vi "Initialize Custom Device Settings.vi"(8 "error in":errorcluster, 10 "Compiled Settings":variant, 11 "Engine Settings in":T2) -> (0 "error out":errorcluster, 1 "ChannelRefs":T1, 3 "Engine Settings out":T2)   [LabVIEW 2026, in "SystemMonitor Engine.lvlib" / "SystemMonitor Engine.lvclass"]
uses:
  SystemMonitor Engine.lvclass
  Types/TargetSettings.ctl
  Shared/GroupedChannelRefs.ctl
  Shared/Compiled.Settings.ctl
  Shared/CustomDeviceSettings.ctl
  Shared/ChannelGroups.ctl
  Shared/GroupSettings.ctl
  Shared/GroupedChannel.ctl
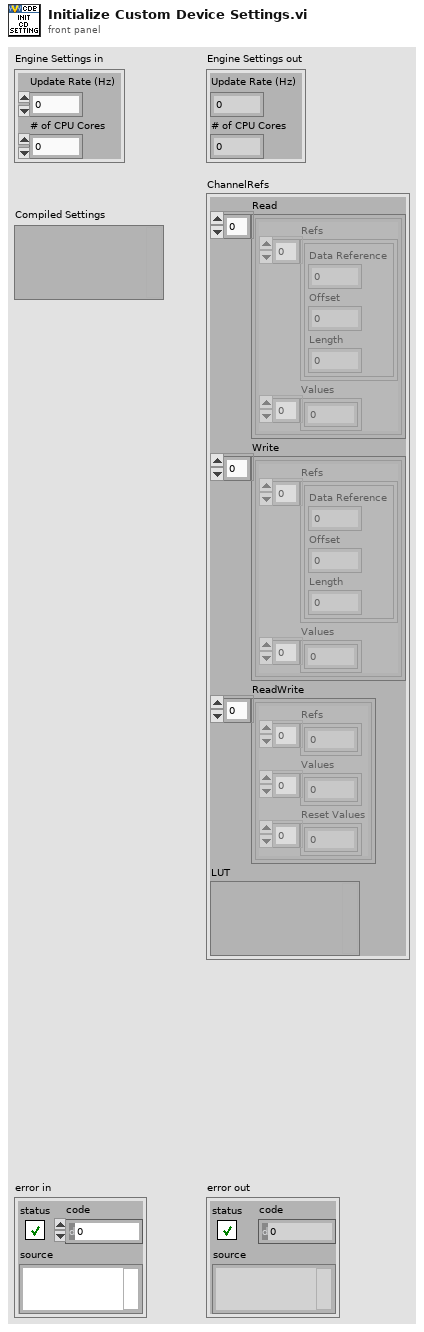
[diagram p1: front panel]
types:
  T1 = typedef "GroupedChannelRefs.ctl" = cluster{"Read":cluster{"Refs":cluster{"Data Reference":i32, "Offset":u64, "Length":u64}[], "Values":dbl[]}[], "Write":cluster{"Refs":cluster{"Data Reference":i32, "Offset":u64, "Length":u64}[], "Values":dbl[]}[], "ReadWrite":cluster{"Refs":i32[], "Values":dbl[], "Reset Values":dbl[]}[], "LUT":variant}
  T2 = typedef "SystemMonitor Engine.lvlib/SystemMonitor Engine.lvclass/TargetSettings.ctl" = cluster{"Update Rate (Hz)":dbl, "# of CPU Cores":i32}
  T3 = typedef "Compiled.Settings.ctl" = cluster{"SystemMonitor":T4, "Channel Groups":T5}
  T4 = typedef "CustomDeviceSettings.ctl" = cluster{"Name":string, "Properties":cluster{"Update Rate (Hz)":dbl, "TargetOS":string, "TargetRate":dbl}, "Sections":cluster{"CPUOverall[]":cluster{"Name":string, "Channels":cluster{"AverageType[]":cluster{"Name":string, "DefaultValue":dbl, "Units":string, "GroupName":string, "Type":string, "Faultable":bool, "Scalable":bool, "ChannelDataReference":i32, "GroupIndex":i32}[], "MaximumType[]":cluster{"Name":string, "DefaultValue":dbl, "Units":string, "GroupName":string, "Type":string, "Faultable":bool, "Scalable":bool, "ChannelDataReference":i32, "GroupIndex":i32}[]}}[], "MemoryUsage[]":cluster{"Name":string, "Channels":cluster{"TotalMemoryType[]":cluster{"Name":string, "DefaultValue":dbl, "Units":string, "GroupName":string, "Type":string, "Faultable":bool, "Scalable":bool, "ChannelDataReference":i32, "GroupIndex":i32}[], "AvailableType[]":cluster{"Name":string, "DefaultValue":dbl, "Units":string, "GroupName":string, "Type":string, "Faultable":bool, "Scalable":bool, "ChannelDataReference":i32, "GroupIndex":i32}[]}}[], "CPU[]":cluster{"Name":string, "Channels":cluster{"TotalType[]":cluster{"Name":string, "DefaultValue":dbl, "Units":string, "GroupName":string, "Type":string, "Faultable":bool, "Scalable":bool, "ChannelDataReference":i32, "GroupIndex":i32}[], "TimeCriticalType[]":cluster{"Name":string, "DefaultValue":dbl, "Units":string, "GroupName":string, "Type":string, "Faultable":bool, "Scalable":bool, "ChannelDataReference":i32, "GroupIndex":i32}[], "TimedStructuresType[]":cluster{"Name":string, "DefaultValue":dbl, "Units":string, "GroupName":string, "Type":string, "Faultable":bool, "Scalable":bool, "ChannelDataReference":i32, "GroupIndex":i32}[], "HighType[]":cluster{"Name":string, "DefaultValue":dbl, "Units":string, "GroupName":string, "Type":string, "Faultable":bool, "Scalable":bool, "ChannelDataReference":i32, "GroupIndex":i32}[], "AboveNormalType[]":cluster{"Name":string, "DefaultValue":dbl, "Units":string, "GroupName":string, "Type":string, "Faultable":bool, "Scalable":bool, "ChannelDataReference":i32, "GroupIndex":i32}[], "NormalType[]":cluster{"Name":string, "DefaultValue":dbl, "Units":string, "GroupName":string, "Type":string, "Faultable":bool, "Scalable":bool, "ChannelDataReference":i32, "GroupIndex":i32}[], "BackgroundType[]":cluster{"Name":string, "DefaultValue":dbl, "Units":string, "GroupName":string, "Type":string, "Faultable":bool, "Scalable":bool, "ChannelDataReference":i32, "GroupIndex":i32}[], "IdleType[]":cluster{"Name":string, "DefaultValue":dbl, "Units":string, "GroupName":string, "Type":string, "Faultable":bool, "Scalable":bool, "ChannelDataReference":i32, "GroupIndex":i32}[], "ISRType[]":cluster{"Name":string, "DefaultValue":dbl, "Units":string, "GroupName":string, "Type":string, "Faultable":bool, "Scalable":bool, "ChannelDataReference":i32, "GroupIndex":i32}[]}}[]}}
  T5 = typedef "ChannelGroups.ctl" = cluster{"Channel Refs":T1, "Group Settings":T6[]}
  T6 = typedef "GroupSettings.ctl" = cluster{"Name":string, "Type":enum16{"Output/Write", "Input/Read", "Input/ReadWrite"}, "Channel Settings":T7[]}
  T7 = typedef "GroupedChannel.ctl" = cluster{"Name":string, "TypeName":string, "ChannelProperties":variant}
  T8 = cluster{"Name":string, "Channels":cluster{"TotalType[]":cluster{"Name":string, "DefaultValue":dbl, "Units":string, "GroupName":string, "Type":string, "Faultable":bool, "Scalable":bool, "ChannelDataReference":i32, "GroupIndex":i32}[], "TimeCriticalType[]":cluster{"Name":string, "DefaultValue":dbl, "Units":string, "GroupName":string, "Type":string, "Faultable":bool, "Scalable":bool, "ChannelDataReference":i32, "GroupIndex":i32}[], "TimedStructuresType[]":cluster{"Name":string, "DefaultValue":dbl, "Units":string, "GroupName":string, "Type":string, "Faultable":bool, "Scalable":bool, "ChannelDataReference":i32, "GroupIndex":i32}[], "HighType[]":cluster{"Name":string, "DefaultValue":dbl, "Units":string, "GroupName":string, "Type":string, "Faultable":bool, "Scalable":bool, "ChannelDataReference":i32, "GroupIndex":i32}[], "AboveNormalType[]":cluster{"Name":string, "DefaultValue":dbl, "Units":string, "GroupName":string, "Type":string, "Faultable":bool, "Scalable":bool, "ChannelDataReference":i32, "GroupIndex":i32}[], "NormalType[]":cluster{"Name":string, "DefaultValue":dbl, "Units":string, "GroupName":string, "Type":string, "Faultable":bool, "Scalable":bool, "ChannelDataReference":i32, "GroupIndex":i32}[], "BackgroundType[]":cluster{"Name":string, "DefaultValue":dbl, "Units":string, "GroupName":string, "Type":string, "Faultable":bool, "Scalable":bool, "ChannelDataReference":i32, "GroupIndex":i32}[], "IdleType[]":cluster{"Name":string, "DefaultValue":dbl, "Units":string, "GroupName":string, "Type":string, "Faultable":bool, "Scalable":bool, "ChannelDataReference":i32, "GroupIndex":i32}[], "ISRType[]":cluster{"Name":string, "DefaultValue":dbl, "Units":string, "GroupName":string, "Type":string, "Faultable":bool, "Scalable":bool, "ChannelDataReference":i32, "GroupIndex":i32}[]}}[]
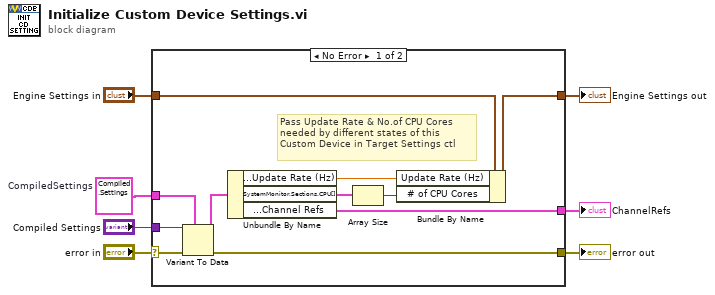
[diagram p0: block diagram]
diagram:
  w2 = T3 {"SystemMonitor"={"Name"="", "Properties"={"Update Rate (Hz)"=0.0, "TargetOS"="", "TargetRate"=0.0}, "Sections"={"CPUOverall[]"=[], "MemoryUsage[]"=[], "CPU[]"=[]}}, "Channel Groups"={"Channel Refs"={"Read"=[], "Write"=[], "ReadWrite"=[], "LUT"=variant}, "Group Settings"=[]}}  # CompiledSettings
  n1 = case shown="No Error" "error in" {
    selector: "error in" -> [w18 w20]
    tunnel: [w17 w20] -> w6
    tunnel: [w11 w19] -> w5
    tunnel: "Engine Settings in" -> [w12 w19]
    tunnel: "Compiled Settings" -> [w16 _]
    tunnel: w2 -> [w15 _]
    tunnel: [w8 _] -> w1
    frame No Error {
      # "Pass Update Rate & No.of CPU Cores\nneeded by different states of this\nCustom Device in Target Settings ctl"
      n2 = Variant To Data(error in=w18, type=w15, Variant=w16) -> (data=w14:T3, error out=w17:errorcluster)
      n3 = Unbundle By Name(w14) -> ("SystemMonitor.Properties.Update Rate (Hz)"=w10:dbl, "SystemMonitor.Sections.CPU[]"=w13:T8, "Channel Groups.Channel Refs"=w8:T1)
      n4 = Array Size(array=w13) -> (size(s)=w9:i32)
      n5 = Bundle By Name(cluster=w12, "Update Rate (Hz)"=w10, "# of CPU Cores"=w9) -> (w11:T2)
    }
    frame Error {
    }
  }
  "error out" <- w6
  "Engine Settings out" <- w5
  "ChannelRefs" <- w1
